vi "Get State From Value.vi"(8 "error in (no error)":errorcluster, 10 "Container State":T4, 11 "Display State In 2":T5 caption="State") -> (0 "error out":errorcluster, 2 "Waveform State":T1={"Show Axes"=FALSE, "Show Y=0"=FALSE, "Controls"={"Type"=enum."Sine", "Periods"=0.0, "Points"=0, "Offset"=0.0, "Amplitdue"=0.0, "Phase"=0.0, "func"=""}, "Show Current Location"=FALSE, "Current Location"=0, "dt"=0.0, "t0"=timestamp(0 s since 1904-01-01), "Format and Units"="%_3p"} caption="State", 3 "Display State In":T5 caption="State")   [LabVIEW 2018]
uses:
  Waveform Control.xctl
  Function Types.ctl
  FP Controls.ctl
  Controls/State.ctl
  <vilib>/_xctls/Container State.ctl
  <vilib>/_xctls/XControlSupport.lvlib
  Controls/Waveform State.ctl
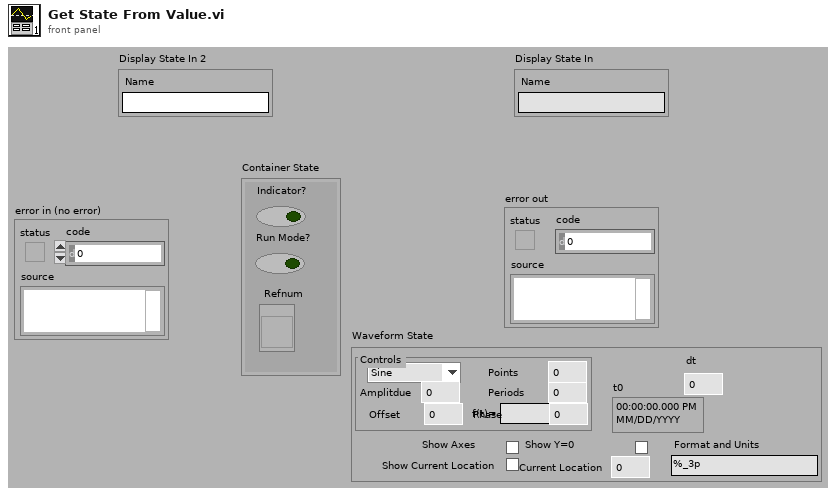
[diagram p1: front panel]
types:
  T1 = typedef "Waveform Control.xctl/Waveform State.ctl" = cluster{"Show Axes":bool, "Show Y=0":bool, "Controls":T2, "Show Current Location":bool, "Current Location":i32, "dt":dbl, "t0":timestamp, "Format and Units":string}
  T2 = typedef "Waveform Control.xctl/FP Controls.ctl" = cluster{"Type":T3, "Periods":dbl, "Points":i32, "Offset":dbl, "Amplitdue":dbl, "Phase":dbl, "func":string}
  T3 = typedef "Waveform Control.xctl/Function Types.ctl" = enum16{"Level", "Sine", "Triangle", "Ramp", "Saw Tooth", "Square", "Function"}
  T4 = typedef "XControlSupport.lvlib/Container State.ctl" = cluster{"Indicator?":bool, "Run Mode?":bool, " Refnum":refnum<vi>}
  T5 = typedef "Waveform Control.xctl/State.ctl" = cluster{"Name":string}
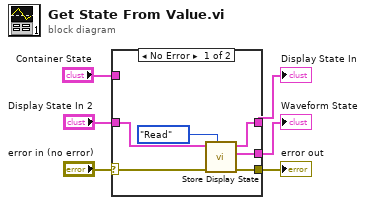
[diagram p0: block diagram]
diagram:
  n1 = case shown="No Error" "error in (no error)" {
    selector: "error in (no error)" -> [w7 w14]
    tunnel: "Container State" -> [_ _]
    tunnel: "Display State In 2" -> [w8 w13]
    tunnel: [w12 w13] -> w3
    tunnel: [w11 w14] -> w2
    tunnel: [w9 _] -> w1
    frame No Error {
      n2 = call "Store Display State.vi"("Operation In"=enum16{"Read", "Write"}."Read" ("Operation"), "Error In (no Error) In"=w7, "State In"=w8) -> ("Error Out"=w11:errorcluster, "Waveform State Out"=w9:T1, "Display State Out"=w12:T5)  [unwired: 3 in, 3 out]
    }
    frame Error {
    }
  }
  "Display State In" <- w3
  "error out" <- w2
  "Waveform State" <- w1
